vi "LoadVIsFromFolder.vi"(8 "error in (no error)":errorcluster, 11 "FolderPath":path) -> (0 "error out":errorcluster, 3 "VIs":refnum<vi>[](array[refnum]))   [LabVIEW 2020]
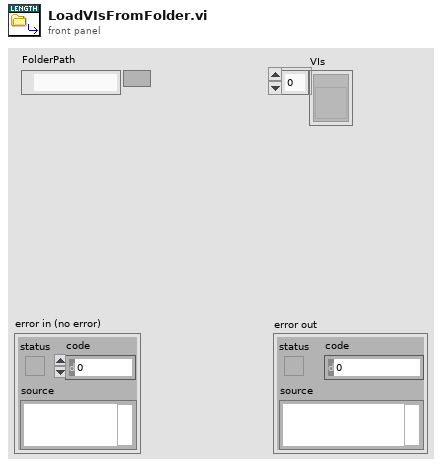
[diagram p1: front panel]
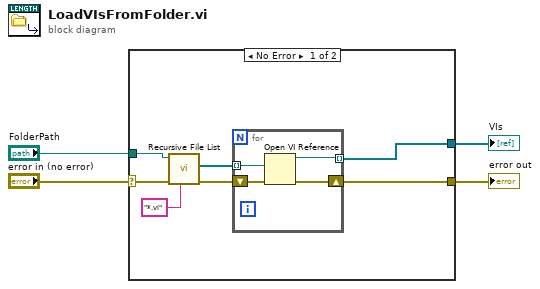
[diagram p0: block diagram]
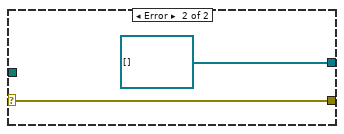
[diagram p2: hidden frame]
diagram:
  n1 = case shown="No Error" "error in (no error)" {
    selector: "error in (no error)" -> [w11 w17]
    tunnel: [w6 w17] -> w4
    tunnel: "FolderPath" -> [w10 _]
    tunnel: [w5 refnum<vi>[] []] -> w1
    frame No Error {
      n2 = call <vilib>:"Recursive File List.vi"("pattern"="*.vi", "error in (no error)"=w11, "Folder Path"=w10) -> ("error out"=w7:errorcluster, "All Files in Dir"=w8:path[])  [unwired: 4 in, 3 out]
      n3 = for {
        tunnel: w8 -> [w15] mode=indexing
        shift-right: [w13] -> w6
        shift-left: w7 -> [w14]
        tunnel: [w12] -> w5 mode=indexing
        n4 = Open VI Reference(vi path=w15, error in (no error)=w14) -> (vi reference=w12:refnum<vi>, error out=w13:errorcluster)  [unwired: 4 in]
      }
    }
    frame Error {
    }
  }
  "error out" <- w4
  "VIs" <- w1
